vi "CalculoOndaPontos.vi"(8 "TimeInicio":u32, 9 "TempoEntrePontos":dbl, 10 "Pontos":dbl[](array[numeric]), 11 "GraphPontos":cluster{"X":dbl, "Y":dbl}[](array[cluster])) -> (0 "Stop":bool, 3 "XY Graph":cluster{"X":dbl, "Y":dbl}[](graph))   [LabVIEW 2019]
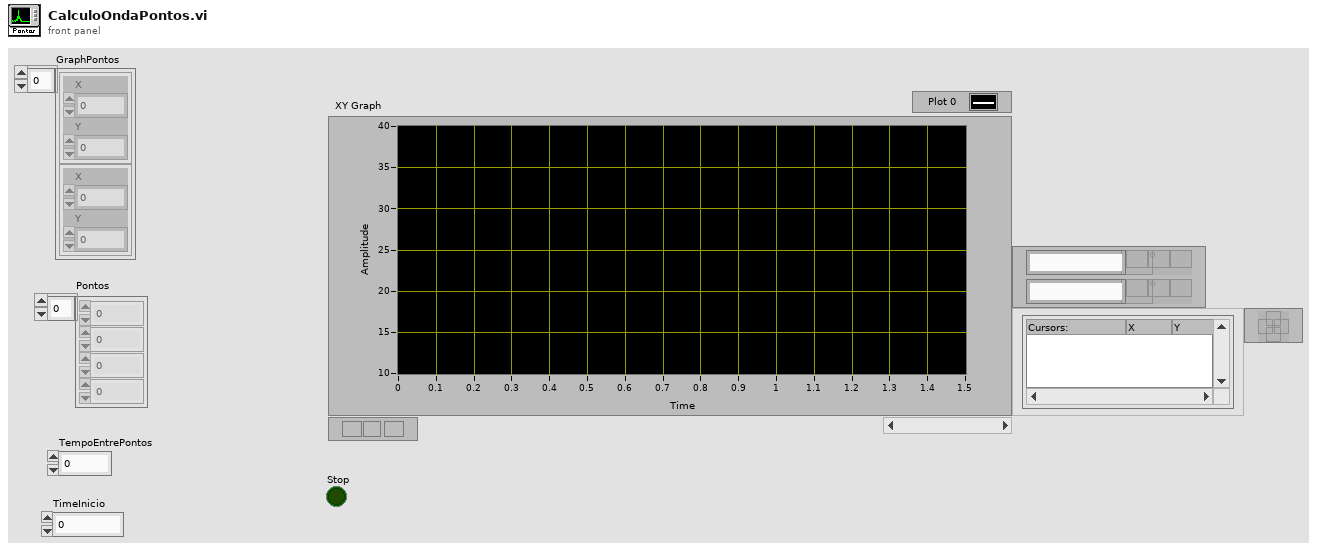
[diagram p1: front panel]
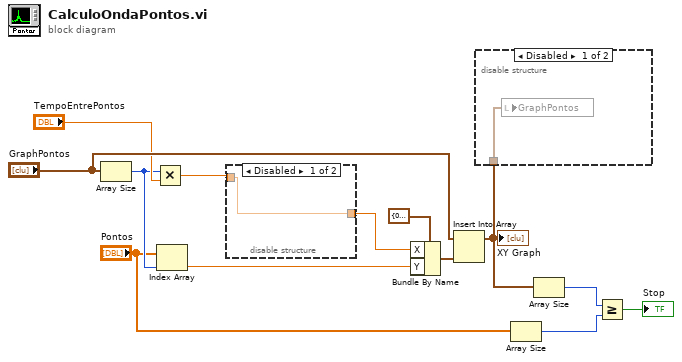
[diagram p0: block diagram]
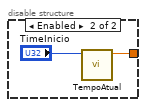
[diagram p2: hidden frame]
diagram:
  n1 = Array Size(array="GraphPontos") -> (size(s)=w9:i32)
  n2 = Multiply(x=w9, y="TempoEntrePontos") -> (x*y=w1:dbl)
  n3 = Index Array(array="Pontos", index=w9) -> (element=w8:dbl)
  n4 = disable-structure shown="Disabled" {
    disable-tunnel: [w14 w15] -> w2
    disable-tunnel: w1 -> [w14 _]
    frame Disabled {
    }
    frame Enabled {
      n5 = call "TempoAtual.vi"("TimeInicio"="TimeInicio") -> ("TempoAtual"=w15:dbl)  [unwired: 10 in]
    }
  }
  n6 = Bundle By Name(cluster=cluster{"X":dbl, "Y":dbl} {"X"=0.0, "Y"=0.0} ("new element/subarray"), "X"=w2, "Y"=w8) -> (w11:cluster{"X":dbl, "Y":dbl})
  n7 = Insert Into Array(array="GraphPontos", new element=w11) -> (w6:cluster{"X":dbl, "Y":dbl}[])  [unwired: 1 in]
  "XY Graph" <- w6
  n8 = disable-structure shown="Disabled" {
    disable-tunnel: w6 -> [w17 _]
    frame Disabled {
      n9 = local write "GraphPontos"(w17) -> ()
    }
    frame Enabled {
    }
  }
  n10 = Array Size(array="Pontos") -> (size(s)=w4:i32)
  n11 = Array Size(array=w6) -> (size(s)=w5:i32)
  n12 = Greater Or Equal?(x=w5, y=w4) -> (x >= y?=→"Stop":bool)
